vi "sensor reading.vi"(1 "Input parameter":T2) -> (0 "readings":T1)   [LabVIEW 2020]
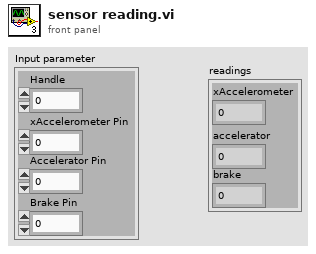
[diagram p1: front panel]
types:
  T1 = cluster{"xAccelerometer":dbl, "accelerator":dbl, "brake":dbl}
  T2 = cluster{"Handle":i32, "xAccelerometer Pin":i32, "Accelerator Pin":i32, "Brake Pin":i32}
  T3 = cluster{"Voltage":dbl, "Voltage":dbl, "Voltage":dbl}
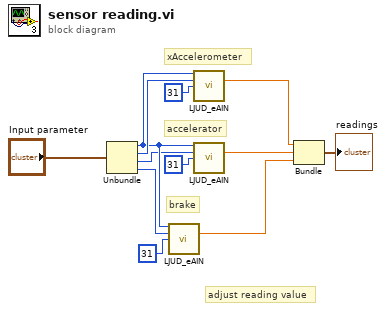
[diagram p0: block diagram]
diagram:
  # "adjust reading value"
  # "brake"
  # "accelerator"
  # "xAccelerometer"
  n1 = Unbundle("Input parameter") -> ("Handle"=w6:i32, "xAccelerometer Pin"=w12:i32, "Accelerator Pin"=w5:i32, "Brake Pin"=w4:i32)
  n2 = call <vilib>:"LJUD_eAIN.vi"("Handle In"=w6, "ChannelP"=w4, "ChannelN"=31) -> ("Voltage"=w1:dbl)  [unwired: 10 in, 2 out]
  n3 = call <vilib>:"LJUD_eAIN.vi"("Handle In"=w6, "ChannelP"=w12, "ChannelN"=31) -> ("Voltage"=w8:dbl)  [unwired: 10 in, 2 out]
  n4 = call <vilib>:"LJUD_eAIN.vi"("Handle In"=w6, "ChannelP"=w5, "ChannelN"=31) -> ("Voltage"=w3:dbl)  [unwired: 10 in, 2 out]
  n5 = Bundle("Voltage"=w8, "Voltage"=w3, "Voltage"=w1) -> (→"readings":T3)  [unwired: 1 in]
